vi "Pre-Build Action - Copy.vi"(6 "Top Level/Always Included VIs":path[](array[path]), 7 "Main Destination Path":path, 9 "Target Name":string, 10 "Build Specification Name":string, 11 "Project Path":path) -> ()   [LabVIEW 2018]
uses:
  <vilib>/Utility/config.llb/NI_LVConfig.lvlib
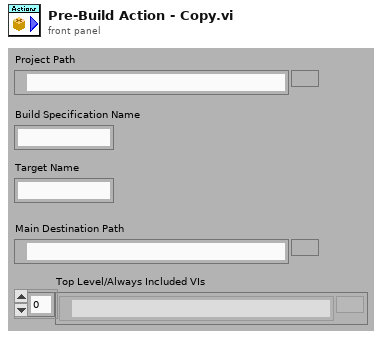
[diagram p1: front panel]
types:
  T1 = typedef "NI_LVConfig.lvlib/Config Data RefNum.ctl" = refnum<k1>
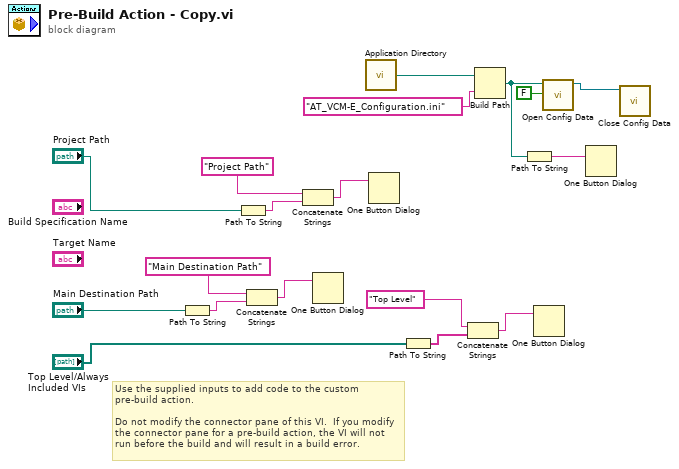
[diagram p0: block diagram]
diagram:
  # "Use the supplied inputs to add code to the custom pre-build action.\n\nDo not modify the connector pane of this VI.  If you modify the connector pane for a pre-build action, the VI will not run before the build and will result in a build error."
  n1 = Path To String(path="Main Destination Path") -> (string=w13:string)
  n2 = Path To String(path="Project Path") -> (string=w8:string)
  n3 = Concatenate Strings("Main Destination Path", w13) -> (w11:string)
  n4 = Concatenate Strings("Project Path", w8) -> (w10:string)
  n5 = One Button Dialog(message=w11) -> ()  [unwired: 1 in, 1 out]
  n6 = call <vilib>:"Application Directory.vi"() -> ("Application Directory"=w18:path)
  n7 = One Button Dialog(message=w10) -> ()  [unwired: 1 in, 1 out]
  n8 = Path To String(path="Top Level/Always Included VIs") -> (string=w6:string[])
  n9 = Concatenate Strings("Top Level", w6) -> (w5:string)
  n10 = Build Path(base path=w18, name or relative path="AT_VCM-E_Configuration.ini") -> (appended path=w3:path)
  n11 = Path To String(path=w3) -> (string=w2:string)
  n12 = One Button Dialog(message=w5) -> ()  [unwired: 1 in, 1 out]
  n13 = call <vilib>:"Open Config Data.vi"("create file if necessary (T)"=FALSE, "configuration file path"=w3) -> ("refnum"=w15:T1)  [unwired: 1 in, 8 out]
  n14 = One Button Dialog(message=w2) -> ()  [unwired: 1 in, 1 out]
  n15 = call <vilib>:"Close Config Data.vi"("refnum"=w15) -> ()  [unwired: 9 in, 2 out]
